vi "Esercitazione 2 - String.vi"() -> ()   [LabVIEW 2018]
panel:
  out "Total Str with replace":string
  out "String Replaced":string
  in  "Replace With":string
  in  "ToSearch":string
  out "Total Str":string
  in  "St2Concatenate":string
  out "Input Length":i32(slide) scale=0.0..10.0
  in  "N Char":i32
  in  "Start Index":i32
  out "Substring":string
  out "Input Length (numeric)":string
  in  "Input":string
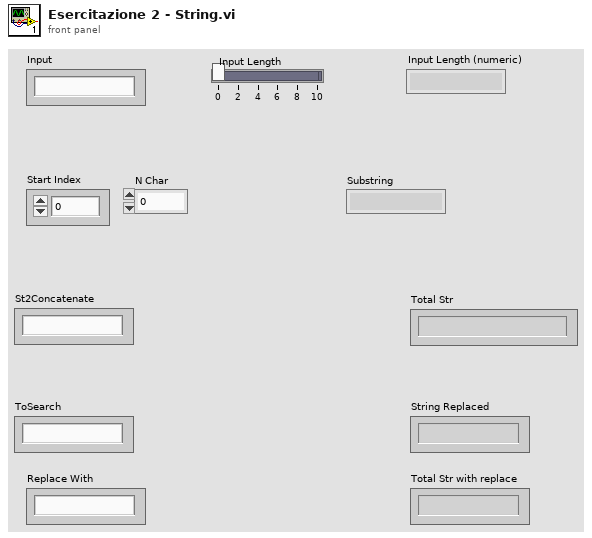
[diagram p1: front panel]
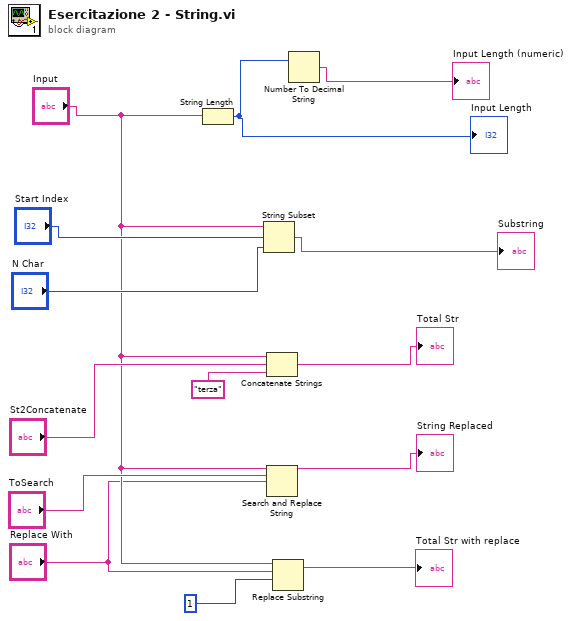
[diagram p0: block diagram]
diagram:
  n1 = String Length(string="Input") -> (length=w10:i32)
  "Input Length" <- w10
  n2 = String Subset(string="Input", offset (0)="Start Index", length (rest)="N Char") -> (substring=→"Substring":string)
  n3 = Concatenate Strings("Input", "St2Concatenate", "terza" ("string")) -> (→"Total Str":string)
  n4 = Search and Replace String(input string="Input", search string="ToSearch", replace string="Replace With") -> (result string=→"String Replaced":string)  [unwired: 5 in, 3 out]
  n5 = Replace Substring(3:1 ("offset (0)"), 4:"Replace With", 5:"Input") -> (1:→"Total Str with replace":string)  [unwired: 1 in, 1 out]
  n6 = Number To Decimal String(number=w10) -> (decimal integer string=→"Input Length (numeric)":string)  [unwired: 1 in]
